vi "Close.vi"(8 "error in":errorcluster, 11 "object in":refnum<class "Scope PXI CFG.lvclass">) -> (0 "error out":errorcluster, 3 "object out":refnum<class "Scope PXI CFG.lvclass">)   [LabVIEW 2023, in "HAL.lvlib" / "Scope PXI.lvlib" / "Scope PXI CFG.lvclass"]
uses:
  Scope PXI CFG.lvclass
  Scope PXI CFG.lvclass/Scope PXI CFG.ctl
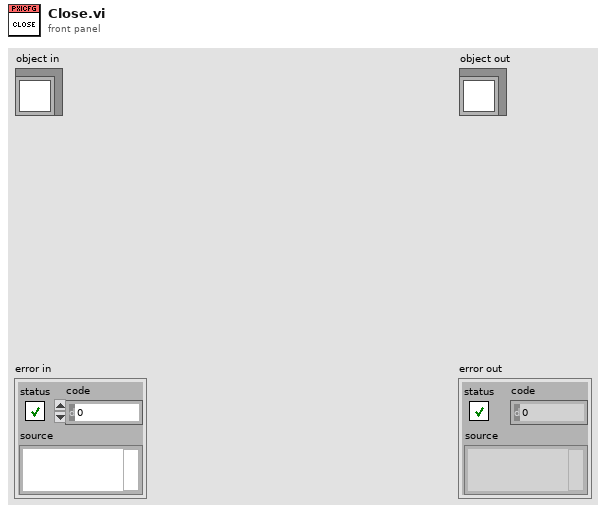
[diagram p1: front panel]
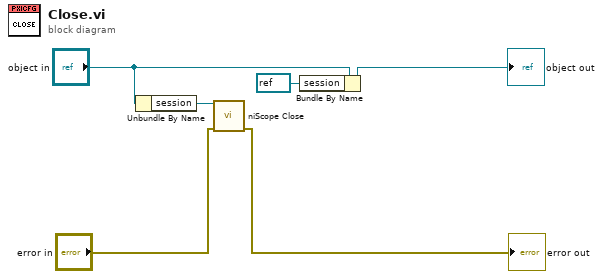
[diagram p0: block diagram]
diagram:
  n1 = Unbundle By Name("object in") -> ("session"=w5:refnum<k15>)
  n2 = call <instrlib>:"niScope Close.vi"("instrument handle"=w5, "error in"="error in") -> ("error out"=→"error out":errorcluster)  [unwired: 13 in]
  n3 = Bundle By Name(cluster="object in", "session"=refnum<k15> refnum) -> (→"object out":refnum<class "Scope PXI CFG.lvclass">)
